vi "Normalize Matrix.vi"(5 "Matrix":T1) -> (0 "error":i32, 1 "mean":dbl format="%0.2f", 2 "standard deviation":dbl format="%0.2f", 3 "Normalized Matrix":T1)   [LabVIEW 2020, in "NI_AALBase.lvlib"]
doc: "Normalizes the input vector or matrix using its statistical profile (micro,s), where micro is the <B>mean</B> and s is the <B>standard deviation</B>, to obtain a <B>Normalized Vector</B> or <B>Normalized Matrix</B> whose statistical profile is (0,1)."
uses:
  NI_AALBase.lvlib
  RealMatrix.ctl
  <resource>/lvanlys.dll
  NI_Matrix.lvlib
panel:
  # "Normalize Matrix"
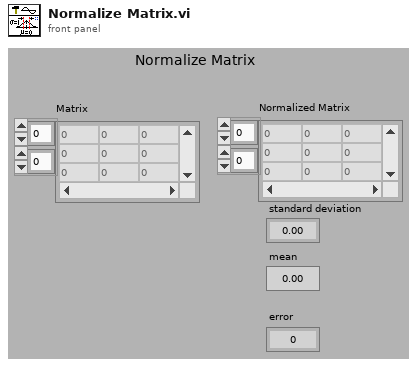
[diagram p1: front panel]
types:
  T1 = typedef "NI_Matrix.lvlib/RealMatrix.ctl" = dbl[][]
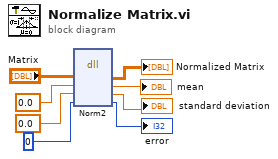
[diagram p0: block diagram]
diagram:
  n1 = dll-call lib="C:/Program Files (x86)/National Instruments/LabVIEW 2020/resource/lvanlys.*" fn="Norm2"("Matrix"="Matrix", 0.0, 0.0, 0) -> ("Matrix"=→"Normalized Matrix":T1, →"mean":dbl, →"standard deviation":dbl, →"error":i32)  [unwired: 4 in, 2 out]
